vi "DriveForDistance-C.vi"(11 "Params":string[][](array[string])) -> ()   [LabVIEW 2017]
uses:
  RoutineData.vi
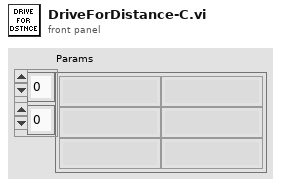
[diagram p1: front panel]
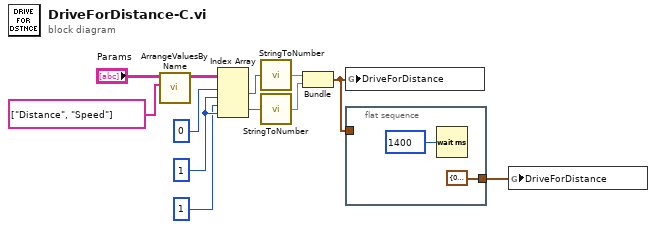
[diagram p0: block diagram]
diagram:
  w4 = 1
  n1 = call "ArrangeValuesByName.vi"("Names"=string[] ["Distance", "Speed"], "Names/Values in"="Params") -> ("Names/Values Out"=w6:string[][])  [unwired: 9 in]
  n2 = Index Array(array=w6, index (row) #1=0, index (col) #1=w4, index (row) #2=1, index (col) #2=w4) -> (element #1=w2:string, element #2=w1:string)
  n3 = call "StringToNumber.vi"("String"=w2) -> ("Output"=w12:dbl)
  n4 = call "StringToNumber.vi"("String"=w1) -> ("Output"=w11:dbl)
  n5 = Bundle("Output"=w12, "Output"=w11) -> (w10:cluster{"Output":dbl, "Output":dbl})  [unwired: 1 in]
  n6 = global write "RoutineData.vi" "DriveForDistance"(w10) -> ()
  n7 = flat-sequence {
    tunnel: w10 -> [_]
    tunnel: [cluster{"Distance":dbl, "Speed":dbl} {"Distance"=0.0, "Speed"=0.0} ("output cluster")] -> w9
    frame #0 {
      n8 = Wait (ms)(milliseconds to wait=u32 1400) -> ()  [unwired: 1 out]
    }
  }
  n9 = global write "RoutineData.vi" "DriveForDistance"(w9) -> ()
